vi "Sequence.BuildWaveformStep.vi"(9 "Current Waveform":waveform(dbl)[](array[waveform]), 10 "Steps":string[](array[string]), 11 "DataPoints":u64) -> (0 "Step Type":T1[](array[typedef]), 1 "IO Points":cluster{"Ramp Pattern":dbl[]}[](array[cluster]), 2 "iStep":bool, 3 "iStep Size":i32)   [LabVIEW 2013, in "Simple Sequence Tools - Shared.lvlib"]
uses:
  Simple Sequence Tools - Shared.lvlib
  Types/Step.Types.ctl
  <vilib>/Analysis/1siggen.llb/Ramp Pattern by Samples.vi
  <vilib>/Analysis/NI_AALBase.lvlib
  <vilib>/measure/NI_MABase.lvlib
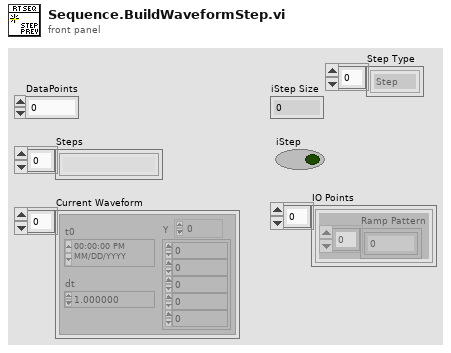
[diagram p1: front panel]
types:
  T1 = typedef "Simple Sequence Tools - Shared.lvlib/Step.Types.ctl" = enum8{"Step", "iStep", "Ramp", "Unchanged", "Unknown", "Sine", "LogSine", "LinearSine", "ForcedRamp", "SquareWave"}
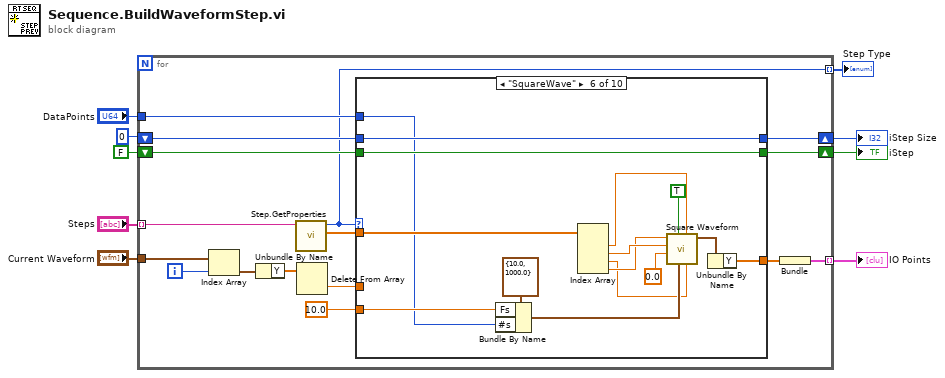
[diagram p0: block diagram]
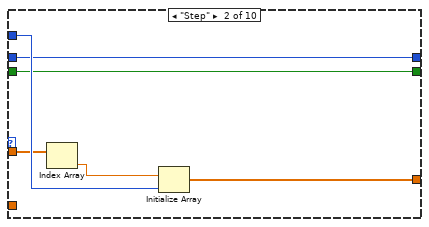
[diagram p3: hidden frame]
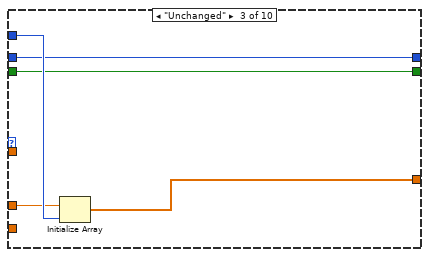
[diagram p4: hidden frame]
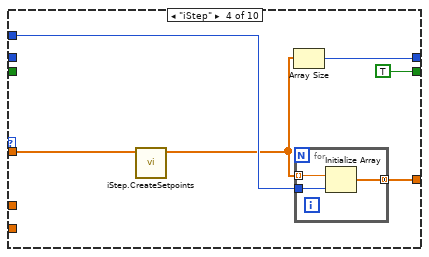
[diagram p5: hidden frame]
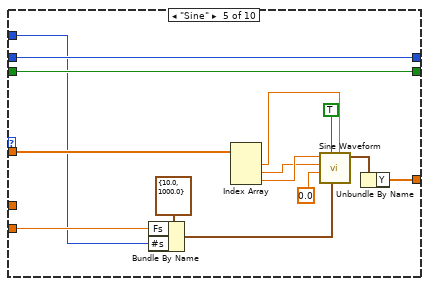
[diagram p6: hidden frame]
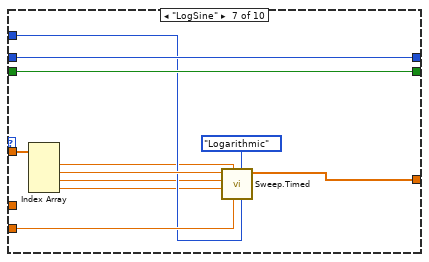
[diagram p7: hidden frame]
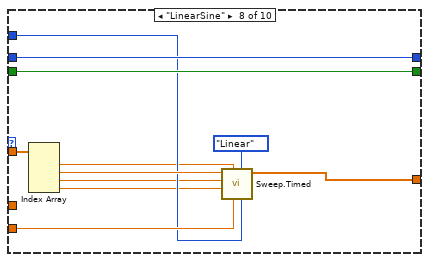
[diagram p8: hidden frame]
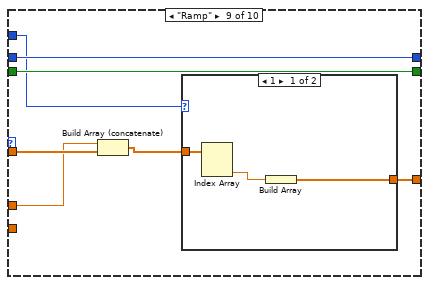
[diagram p9: hidden frame]
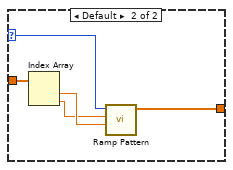
[diagram p10: hidden frame]
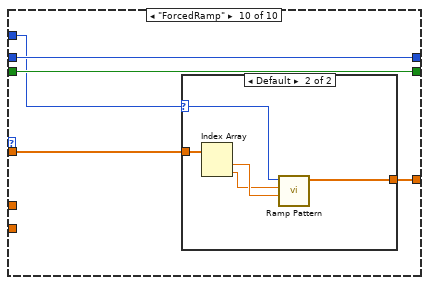
[diagram p11: hidden frame]
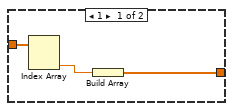
[diagram p12: hidden frame]
diagram:
  n1 = for {
    tunnel: "Steps" -> [w25] mode=indexing
    tunnel: "DataPoints" -> [w24]
    shift-right: [w21] -> w5
    shift-left: FALSE -> [w22]
    shift-right: [w19] -> w6
    shift-left: 0 -> [w18]
    tunnel: [w17] -> w7 mode=indexing
    tunnel: "Current Waveform" -> [w16]
    tunnel: [w10] -> w1 mode=indexing
    i -> [w14]
    n2 = Index Array(array=w16, index=w14) -> (element=w13:waveform(dbl))
    n3 = Unbundle By Name(w13) -> ("Y"=w12:dbl[])
    n4 = call "Step.GetProperties.vi"("String in"=w25) -> ("Parameters"=w23:dbl[], "Step"=w10:T1)  [unwired: 8 in, 1 out]
    n5 = Delete From Array(array=w12) -> (deleted portion=w15:dbl)  [unwired: 2 in, 1 out]
    n6 = case shown="\"SquareWave\"" w10 {
      tunnel: w24 -> [_ w33 w38 w43 w48 w64 w81 w92 w102 w115]
      tunnel: w23 -> [_ w32 _ w44 w61 w76 w85 w96 w101 w114]
      tunnel: [_ w30 w37 w41 w55 w71 w82 w93 w105 w118] -> w20
      tunnel: w22 -> [w27 w29 w36 _ w50 w66 w86 w97 w104 w117]
      tunnel: [w27 w29 w36 TRUE w50 w66 w86 w97 w104 w117] -> w21
      tunnel: [w26 w28 w35 w39 w60 w75 w87 w98 w103 w116] -> w19
      tunnel: w18 -> [w26 w28 w35 _ w60 w75 w87 w98 w103 w116]
      tunnel: w15 -> [_ _ w34 _ _ _ _ _ w100 _]
      tunnel: 10.0 ("Fs") -> [_ _ _ _ w49 w65 w83 w94 _ _]
      frame Default {
      }
      frame "Step" {
        n7 = Index Array(array=w32) -> (element=w31:dbl)  [unwired: 1 in]
        n8 = Initialize Array(w31, w33) -> (w30:dbl[])
      }
      frame "Unchanged" {
        n9 = Initialize Array(w34, w38) -> (w37:dbl[])
      }
      frame "iStep" {
        n10 = call "iStep.CreateSetpoints.vi"("Parameters"=w44) -> ("iStep Pattern"=w40:dbl[])  [unwired: 9 in, 1 out]
        n11 = Array Size(array=w40) -> (size(s)=w39:i32)
        n12 = for {
          tunnel: w43 -> [w47]
          tunnel: w40 -> [w46] mode=indexing
          tunnel: [w45] -> w41 mode=concatenating
          n13 = Initialize Array(w46, w47) -> (w45:dbl[])
        }
      }
      frame "Sine" {
        n14 = Bundle By Name(cluster=cluster{"Fs":dbl, "#s":dbl} {"Fs"=10.0, "#s"=1000.0} ("sampling info"), "Fs"=w49, "#s"=w48) -> (w53:cluster{"Fs":dbl, "#s":dbl})
        n15 = Index Array(array=w61) -> (element #1=w51:dbl, element #2=w52:dbl, element #3=w59:dbl)  [unwired: 3 in]
        n16 = call <vilib>:"Sine Waveform.vi"("offset"=w51, "sampling info"=w53, "reset signal"=TRUE ("reset phase"), "phase"=0.0 ("phase in"), "amplitude"=w52, "frequency"=w59) -> ("signal out"=w56:waveform(dbl))  [unwired: 4 in, 1 out]
        n17 = Unbundle By Name(w56) -> ("Y"=w55:dbl[])
      }
      frame "SquareWave" {
        n18 = Bundle By Name(cluster=cluster{"Fs":dbl, "#s":dbl} {"Fs"=10.0, "#s"=1000.0} ("sampling info"), "Fs"=w65, "#s"=w64) -> (w69:cluster{"Fs":dbl, "#s":dbl})
        n19 = Index Array(array=w76) -> (element #1=w67:dbl, element #2=w68:dbl, element #3=w62:dbl, element #4=w63:dbl)  [unwired: 4 in]
        n20 = call <vilib>:"Square Waveform.vi"("duty cycle (%)"=w62, "offset"=w67, "sampling info"=w69, "reset signal"=TRUE ("reset phase"), "phase"=0.0 ("phase in"), "amplitude"=w68, "frequency"=w63) -> ("signal out"=w72:waveform(dbl))  [unwired: 3 in, 1 out]
        n21 = Unbundle By Name(w72) -> ("Y"=w71:dbl[])
      }
      frame "LogSine" {
        n22 = Index Array(array=w85) -> (element #1=w80:dbl, element #2=w84:dbl, element #3=w79:dbl, element #4=w78:dbl)  [unwired: 4 in]
        n23 = call "Sweep.Timed.vi"("DataPoints"=w81, "frequency spacing"=enum16{"Linear", "Logarithmic"}."Logarithmic", "Fsample (S/s)"=w83, "Offset"=w80, "EndHz"=w78, "StartHz"=w79, "Amplitude"=w84) -> ("Chirp Data"=w82:dbl[])  [unwired: 3 in, 1 out]
      }
      frame "LinearSine" {
        n24 = Index Array(array=w96) -> (element #1=w91:dbl, element #2=w95:dbl, element #3=w90:dbl, element #4=w89:dbl)  [unwired: 4 in]
        n25 = call "Sweep.Timed.vi"("DataPoints"=w92, "frequency spacing"=enum16{"Linear", "Logarithmic"}."Linear", "Fsample (S/s)"=w94, "Offset"=w91, "EndHz"=w89, "StartHz"=w90, "Amplitude"=w95) -> ("Chirp Data"=w93:dbl[])  [unwired: 3 in, 1 out]
      }
      frame "Ramp" {
        n26 = Build Array (concatenate)(w100, w101) -> (w99:dbl[])
        n27 = case shown="1" w102 {
          selector: w102 -> [_ w112]
          tunnel: w99 -> [w108 w111]
          tunnel: [w106 w113] -> w105
          frame 1 {
            n28 = Index Array(array=w108) -> (element #2=w107:dbl)  [unwired: 2 in, 1 out]
            n29 = Build Array(w107) -> (w106:dbl[])
          }
          frame Default {
            n30 = Index Array(array=w111) -> (element #1=w110:dbl, element #2=w109:dbl)  [unwired: 2 in]
            n31 = call-poly <vilib>:"Ramp Pattern.vi"("start"=w110, "end"=w109, "samples"=w112) -> ("Ramp Pattern"=w113:dbl[])  [unwired: 7 in, 1 out]
          }
        }
      }
      frame "ForcedRamp" {
        n32 = case shown="Default" w115 {
          selector: w115 -> [_ w125]
          tunnel: w114 -> [w121 w124]
          tunnel: [w119 w126] -> w118
          frame 1 {
            n33 = Index Array(array=w121) -> (element #2=w120:dbl)  [unwired: 2 in, 1 out]
            n34 = Build Array(w120) -> (w119:dbl[])
          }
          frame Default {
            n35 = Index Array(array=w124) -> (element #1=w123:dbl, element #2=w122:dbl)  [unwired: 2 in]
            n36 = call-poly <vilib>:"Ramp Pattern.vi"("start"=w123, "end"=w122, "samples"=w125) -> ("Ramp Pattern"=w126:dbl[])  [unwired: 7 in, 1 out]
          }
        }
      }
    }
    n37 = Bundle("Ramp Pattern"=w20) -> (w17:cluster{"Ramp Pattern":dbl[]})  [unwired: 1 in]
  }
  "IO Points" <- w7
  "iStep Size" <- w6
  "iStep" <- w5
  "Step Type" <- w1
